vi "testout.vi"() -> ()   [LabVIEW 2013]
uses:
  <vilib>/Platform/TimedLoop/XDataNode/timing_clust.ctl
  <vilib>/Platform/TimedLoop/XDataNode/nitl_modes.ctl
  <vilib>/Platform/TimedLoop/XDataNode/wakeup.ctl
  <vilib>/rvi/Emulation/niFpgaSctlEmulationGetInTimedLoop.vi
  <vilib>/rvi/Emulation/niFpgaEmulationReportErrorSimple.vi
  <vilib>/rvi/Emulation/niFpgaGetClockAttributes.vi
  <vilib>/rvi/eio/common/nirviEmuTemplateMethod_errors.vi
  <vilib>/rvi/Emulation/niFpgaCriticalErrorInLSC.vi
  <vilib>/platform/TimedLoop/XDataNode/XDataNode.xnode
  <vilib>/eio/EIONode/EIONode.xnode
  <vilib>/Platform/TimedLoop/XDataNode/XDNodeRunTimeDep.lvlib
panel:
  in  "stop":bool
  in  "OUTPUT1":bool
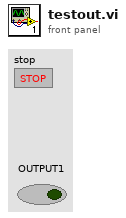
[diagram p1: front panel]
types:
  T1 = typedef "XDNodeRunTimeDep.lvlib/timing_clust.ctl" = cluster{"Expected End [f-1]":u64, "Actual End [f-1]":u64, "Finished Late? [f-1]":bool, "Expected End [i-1]":u64, "Actual End [i-1]":u64, "Finished Late? [i-1]":bool, "Expected Start [i]":u64, "Actual Start [i]":u64, "Expected Start [f]":u64, "Actual Start [f]":u64, "Source Name":string, "Structure Name":string, "Period":i64, "Deadline":i64, "Offset":i64, "Start":i64, "Priority":i32, "Timeout":i32, "Mode":T2, "Wakeup Reason":T3, "Error":errorcluster, "Source Type":string, "Secondary Source Type":string, "Global End Time":u64, "Global Start Time":u64, "Frame Duration":u64, "Iteration Duration":u64, "Assigned CPU":i32, "I/O Scan Engine Mode":u32}
  T2 = typedef "XDNodeRunTimeDep.lvlib/nitl_modes.ctl" = enum32{"No Change", "Process missed periods, maintain original phase", "Discard missed periods, maintain original phase", "Process missed periods, ignore original phase", "Discard missed periods, ignore original phase"}
  T3 = typedef "XDNodeRunTimeDep.lvlib/wakeup.ctl" = enum32{"Normal", "Aborted", "Asynchronous wakeup", "Timing source error", "Timed loop error", "Timeout"}
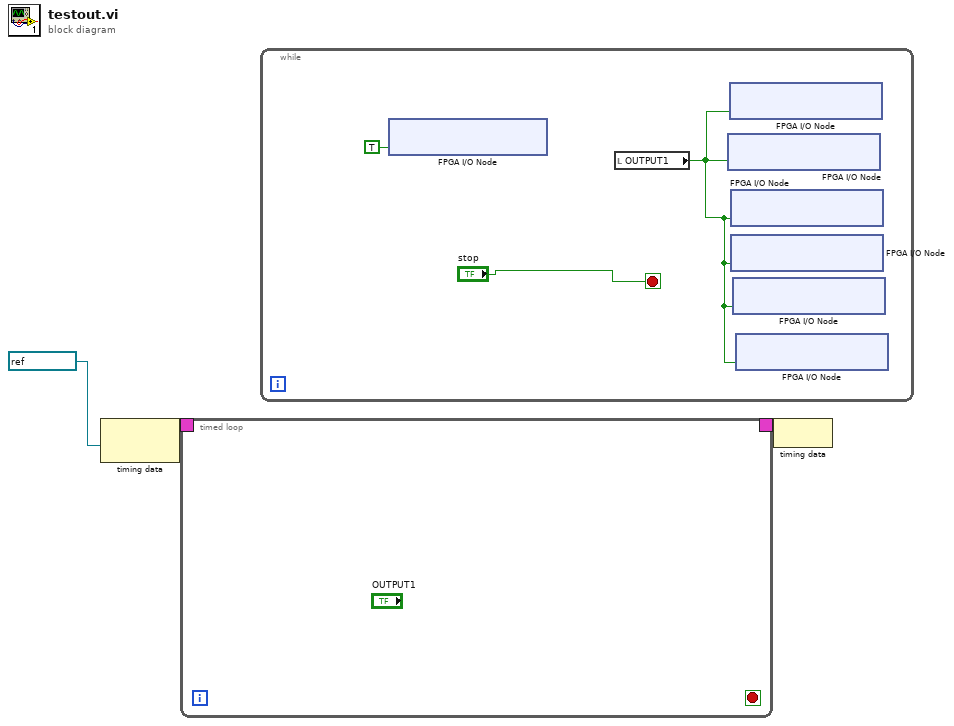
[diagram p0: block diagram]
diagram:
  n1 = node-c288(refnum<k21> "26 MHz" ("Source Name")) -> (w3:T1)
  n2 = timed-loop {
    timing: w3 -> [_]
    timing-out: [_] -> w2
    stop <- _ stop-if-true
  }
  n3 = while {
    stop <- "stop" stop-if-true
    n4 = xnode "FPGA I/O Node"("IO Module\\PFI Enable"=TRUE ("IO Module\\PFI Enable")) -> ()  [unwired: 1 in, 1 out]
    n5 = local read "OUTPUT1"() -> (w6:bool)
    n6 = xnode "FPGA I/O Node"("IO Module\\PFI Out 4"=w6) -> ()  [unwired: 1 in, 1 out]
    n7 = xnode "FPGA I/O Node"("IO Module\\PFI Out 1"=w6) -> ()  [unwired: 1 in, 1 out]
    n8 = xnode "FPGA I/O Node"("IO Module\\PFI Out 2"=w6) -> ()  [unwired: 1 in, 1 out]
    n9 = xnode "FPGA I/O Node"("IO Module\\PFI Out 3"=w6) -> ()  [unwired: 1 in, 1 out]
    n10 = xnode "FPGA I/O Node"("IO Module\\PFI Out 6"=w6) -> ()  [unwired: 1 in, 1 out]
    n11 = xnode "FPGA I/O Node"("IO Module\\PFI Out 7"=w6) -> ()  [unwired: 1 in, 1 out]
  }
  n12 = node-c288(w2) -> ()
